vi "Client 1 JKI SM or SMO.vi"(4 "Enum 2":enum16{"SMO", "Stand Alone"}(ring)=enum."Stand Alone", 6 "Enum":enum16{"RemoteControl", "RemoteControl.STM"}(ring)=enum."RemoteControl.STM", 8 "error in (no error)":errorcluster, 10 "Message to Send":T1) -> (0 "error out":errorcluster, 1 "execution time (ms)":u32, 2 "Message Received":T1)   [LabVIEW 2016, in "RemoteControl.lvclass"]
uses:
  RemoteControl.lvclass
  <vilib>/JKI/JKI SMO/SMO/Typedefs/SMOState --Enum.ctl
  Typedefs/Message--Cluster.ctl
  RemoteControl.STM/RemoteControl.STM.lvclass
  C:/user/patrick/hg/levylab_util_remote/src/SMOs/RemoteControl/RemoteControl.lvclass
  <vilib>/JKI/JKI SMO/SMO/SMO.lvclass
  Typedefs/PrivateEvents--RemoteControl.SendMessageToProcess.ctl
  C:/Program Files (x86)/National Instruments/LabVIEW 2016/vi.lib/JKI/JKI SMO/SMO/SMO.lvclass
panel:
  out "# reads":i32
  out "send time":u32
  in  "timeout in ms (100)":i32=10
  in  "Send Message":bool
  in  "Stop":bool
  out "message backlog":i32
  out "messages received":i32
  out "messages sent":i32
  in  "Port":u32=6341
  in  "Address":string
  out "SMO State":T2
  # "Client 1"
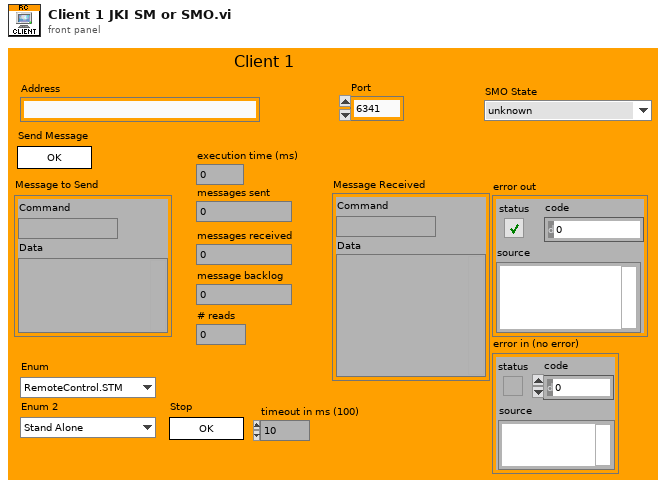
[diagram p1: front panel]
types:
  T1 = typedef "RemoteControl.lvclass/Message--Cluster.ctl" = cluster{"Command":string, "Data":variant}
  T2 = typedef "SMO.lvclass/SMOState --Enum.ctl" = enum16{"unknown", "Created", "Started", "Stopped"}
  T3 = enum32{"Invalid", "Standard", "Closed", "Hidden", "Minimized", "Maximized"}
  T4 = enum32{"invalid app kind", "Development System", "Run Time System", "Student Edition", "Embedded LabVIEW", "Evaluation", "Custom"}
  T5 = typedef "RemoteControl.lvclass/PrivateEvents--RemoteControl.SendMessageToProcess.ctl" = cluster{"Message":T1, "Message ID":u32}
  T6 = cluster{"Core":cluster{"Current VI Reference":refnum<vi>, "Close Panel on Exit?":bool}, "RemoteControl out":refnum<class "RemoteControl.lvclass">}
  T7 = cluster{"Current VI Reference":refnum<vi>, "Close Panel on Exit?":bool}
  T8 = typedef "SMO.lvclass/Public Events.ctl" = cluster{"Error":refnum<user-event>, "State":refnum<user-event>, "Reserve State":refnum<user-event>}
  T9 = typedef "RemoteControl.lvclass/PublicEvents--Cluster.ctl" = cluster{"SendMessageFromProcess":refnum<user-event>}
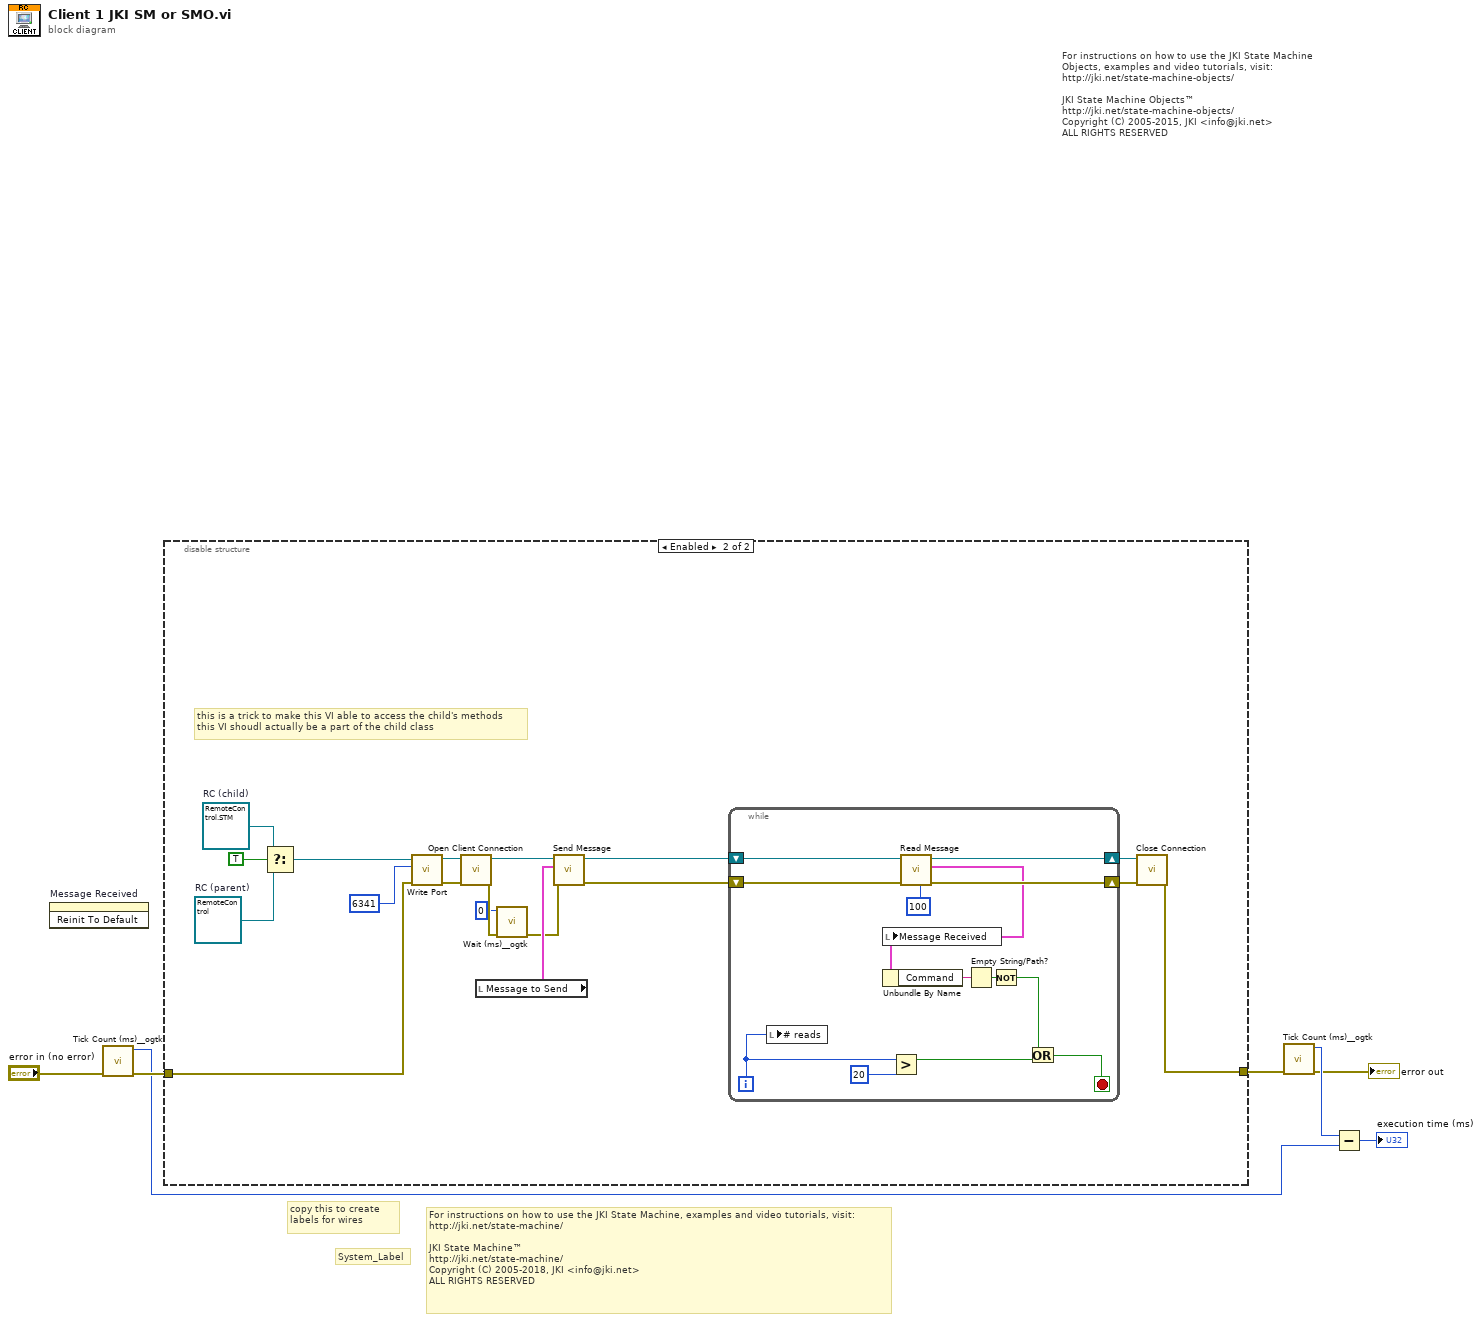
[diagram p0: block diagram]
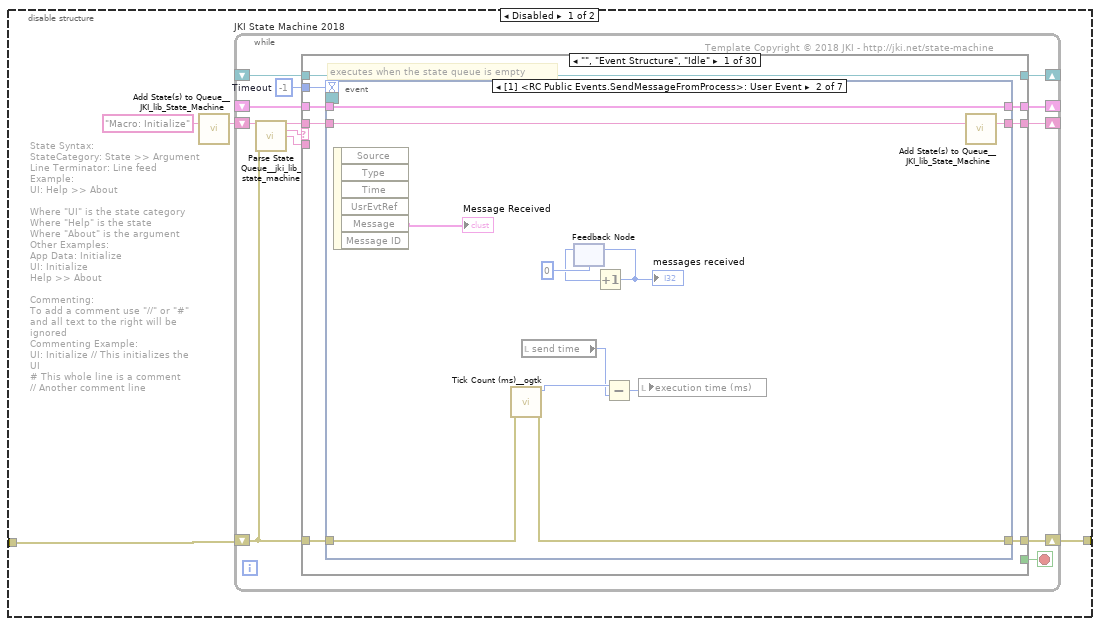
[diagram p2: hidden frame]
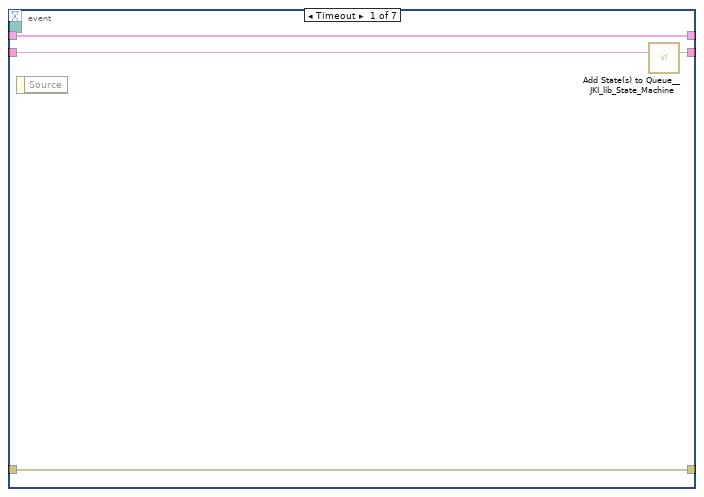
[diagram p3: hidden frame]
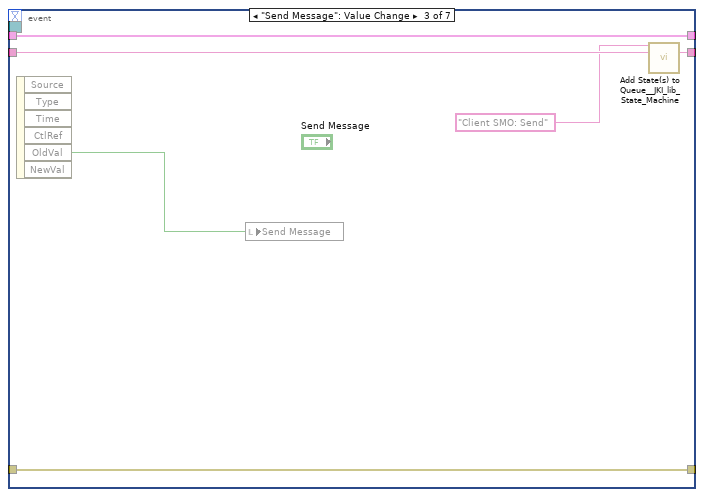
[diagram p4: hidden frame]
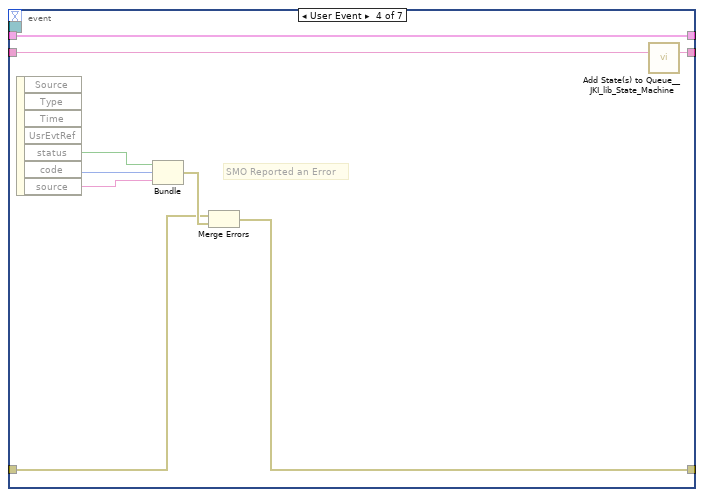
[diagram p5: hidden frame]
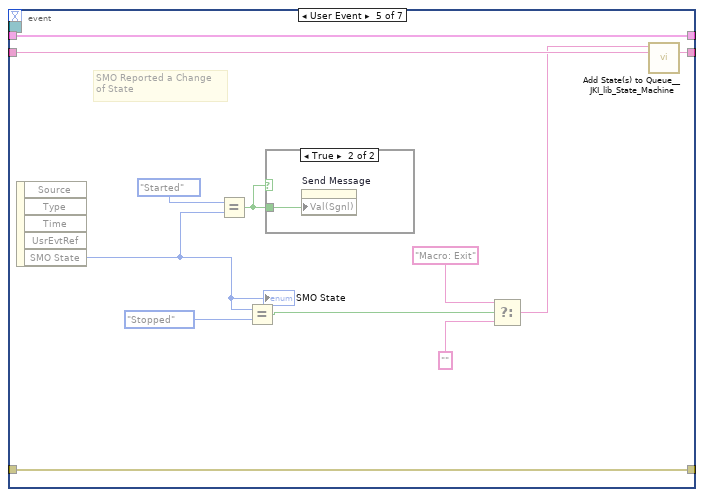
[diagram p6: hidden frame]
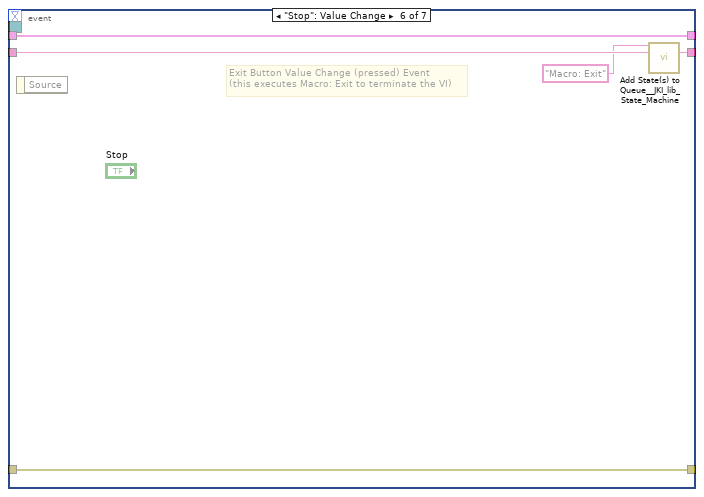
[diagram p8: hidden frame]
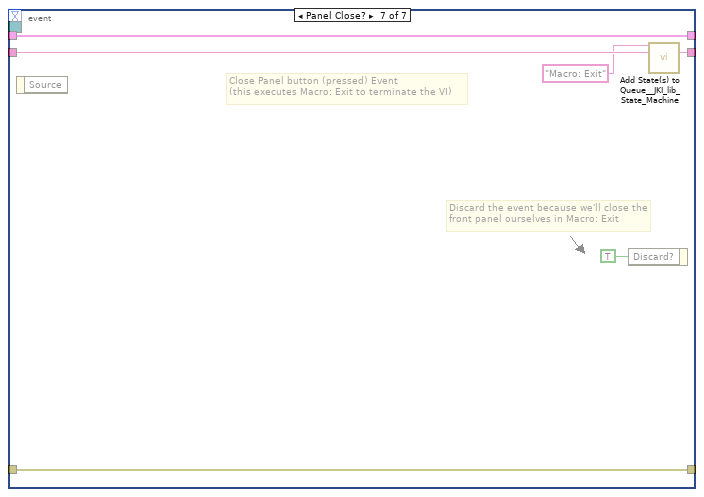
[diagram p9: hidden frame]
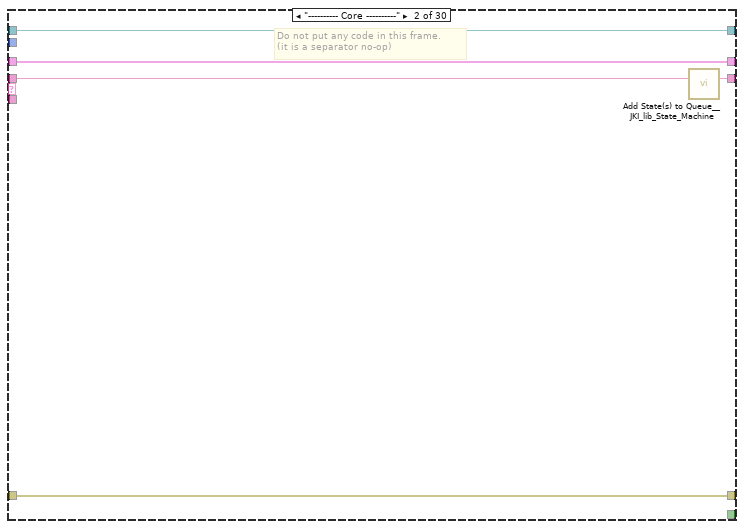
[diagram p10: hidden frame]
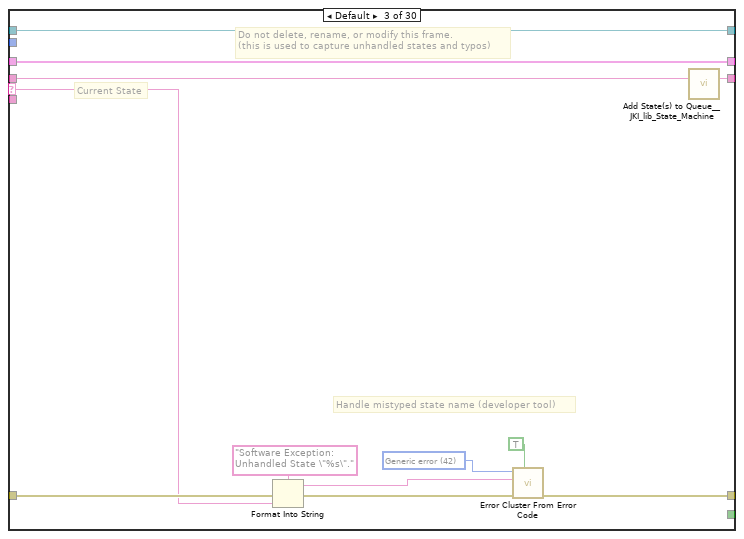
[diagram p11: hidden frame]
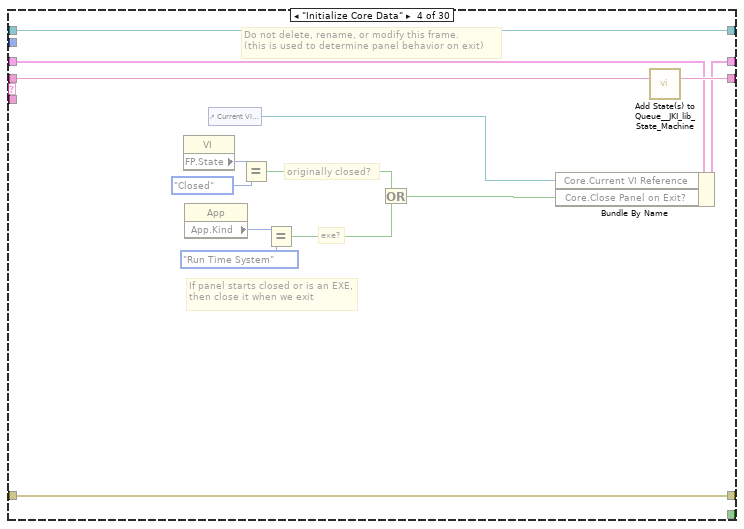
[diagram p12: hidden frame]
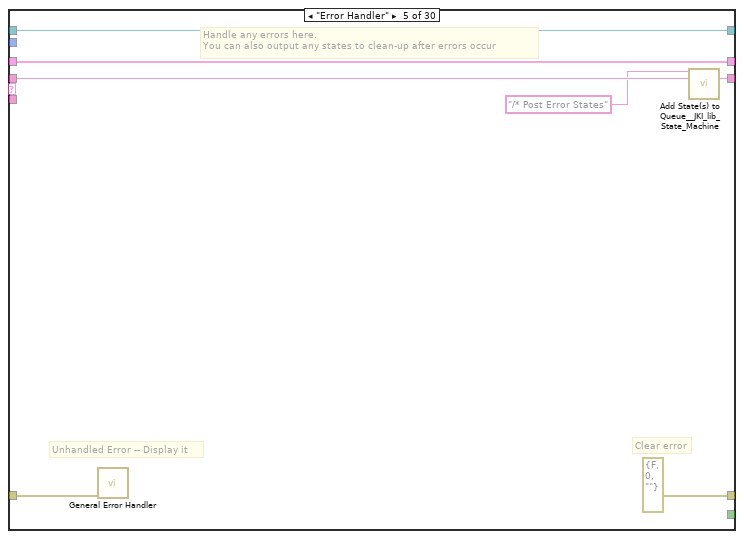
[diagram p13: hidden frame]
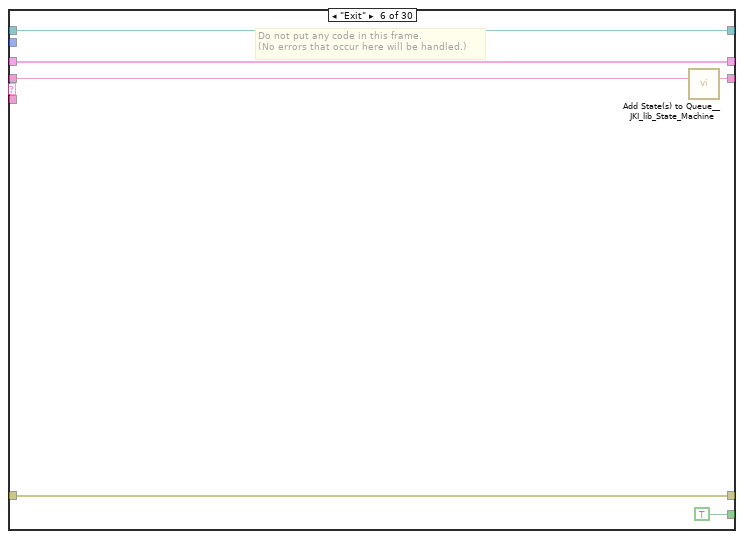
[diagram p14: hidden frame]
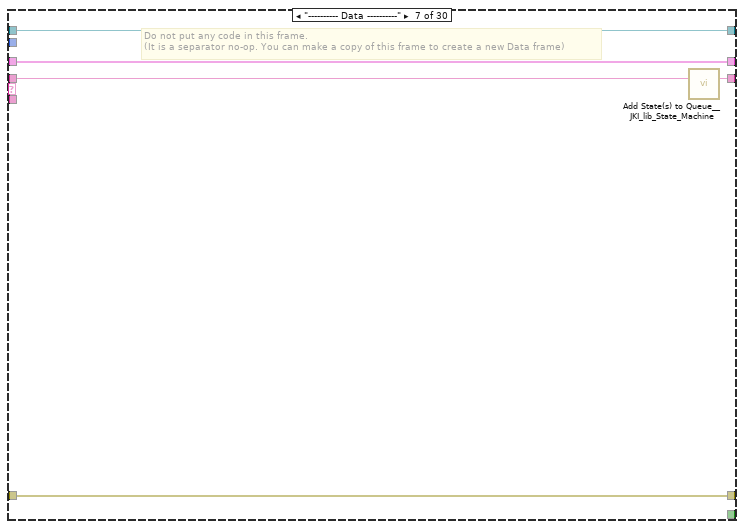
[diagram p15: hidden frame]
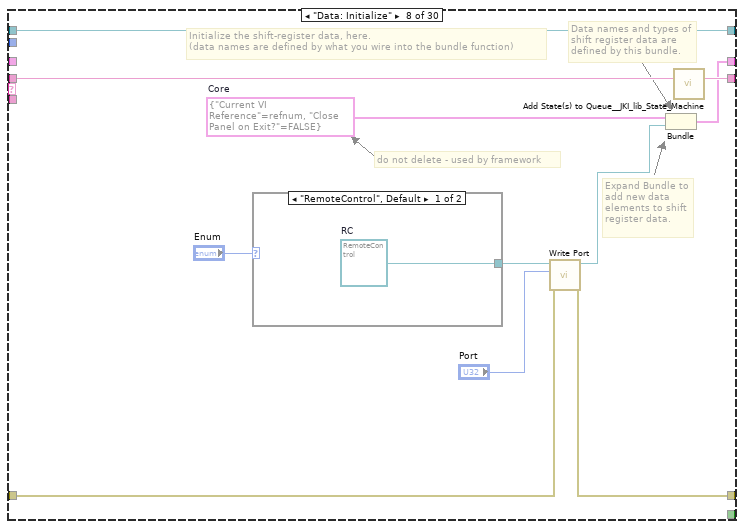
[diagram p16: hidden frame]
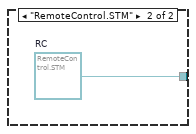
[diagram p17: hidden frame]
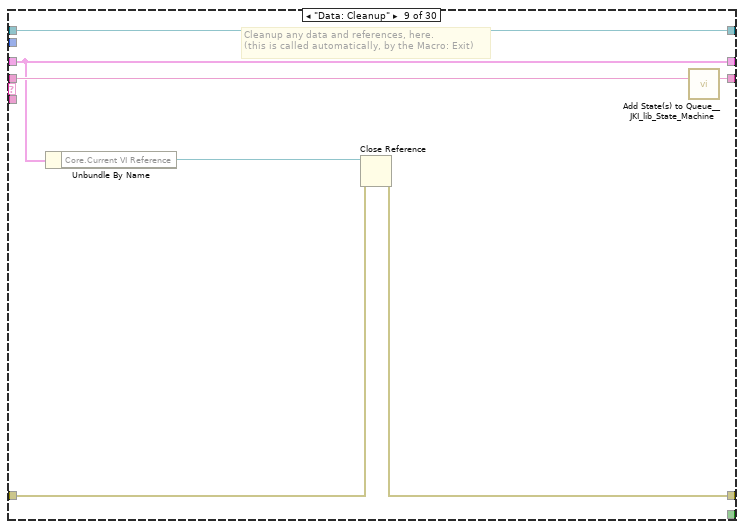
[diagram p18: hidden frame]
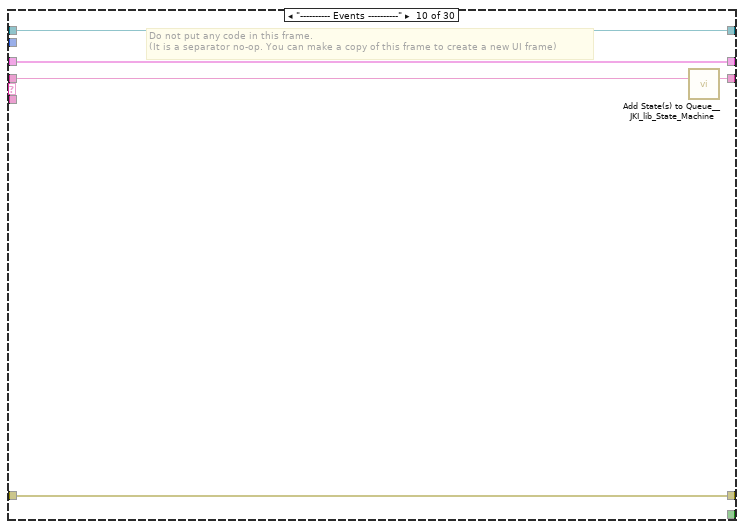
[diagram p19: hidden frame]
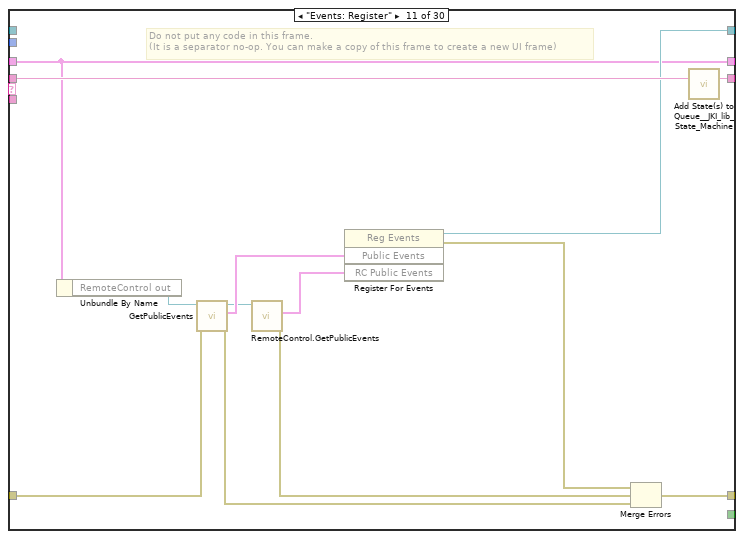
[diagram p20: hidden frame]
diagram:
  # "For instructions on how to use the JKI State Machine, examples and video tutorials, visit:\nhttp://jki.net/state-machine/\n\nJKI State Machine™\nhttp://jki.net/state-machine/\nCopyright (C) 2005-2018, JKI <info@jki.net>\nALL RIGHTS RESERVED"
  # "copy this to create labels for wires"
  # "System_Label"
  # "For instructions on how to use the JKI State Machine Objects, examples and video tutorials, visit:\nhttp://jki.net/state-machine-objects/\n\nJKI State Machine Objects™\nhttp://jki.net/state-machine-objects/\nCopyright (C) 2005-2015, JKI <info@jki.net>\nALL RIGHTS RESERVED"
  n1 = invoke on="Message Received" class="Clust (strict)" method="Reinit To Default"() -> ()  [unwired: 3 in, 3 out]
  n2 = call <userlib>:"Tick Count (ms)__ogtk.vi"("error in (no error)"="error in (no error)") -> ("error out"=w6:errorcluster, "millisecond timer value"=w1:u32)  [unwired: 9 in]
  n3 = disable-structure shown="Enabled" {
    disable-tunnel: w6 -> [w9 w425]
    disable-tunnel: [w8 w424] -> w2
    frame Disabled {
      # "State Syntax:\nStateCategory: State >> Argument\nLine Terminator: Line feed\nExample:\nUI: Help >> About\n\nWhere \"UI\" is the state category\nWhere \"Help\" is the state\nWhere \"About\" is the argument\nOther Examples:\nApp Data: Initialize\nUI: Initialize\nHelp >> About\n\nCommenting:\nTo add a comment use \"//\" or \"#\" and all text to the right will be ignored\nCommenting Example:\nUI: Initialize // This initializes the UI\n# This whole line is a comment\n// Another comment line"
      n4 = call <vilib>:"Add State(s) to Queue__JKI_lib_State_Machine.vi"("State(s) in (\"\")"="Macro: Initialize") -> ("States Out"=w11:string)  [unwired: 14 in]
      n5 = while "JKI State Machine 2018" {
        shift-right: [w17] -> _
        shift-left: _ -> [w16]
        shift-right: [w20] -> w8
        shift-left: w9 -> [w14]
        shift-right: [w19] -> _
        shift-left: w11 -> [w21]
        shift-right: [w13] -> _
        shift-left: _ -> [w12]
        stop <- w18 stop-if-true
        w15 = -1  # Timeout
        # "Template Copyright © 2018 JKI - http://jki.net/state-machine"
        n6 = call <vilib>:"Parse State Queue__jki_lib_state_machine.vi"("State Queue"=w21, "Error In (no error)"=w14) -> ("Remaining States"=w23:string, "Current State"=w24:string, "Arguments"=w22:string)  [unwired: 11 in]
        n7 = case shown="\"\", \"Event Structure\", \"Idle\"" w24 {
          selector: w24 -> [_ _ w94 _ _ _ _ _ _ _ _ _ _ _ _ _ _ _ _ _ _ _ _ _ _ _ _ _ _ _]
          tunnel: w23 -> [w32 w92 w98 w118 w125 w131 w136 w147 w156 w161 w174 w180 w185 w190 w197 w209 w279 w286 w299 w304 w317 w326 w343 w352 w359 w364 w373 w385 w396 w418]
          tunnel: w22 -> [_ _ _ _ _ _ _ _ _ _ _ _ _ _ w192 w203 _ _ _ _ _ _ _ _ _ _ _ _ _ _]
          tunnel: w16 -> [w30 w89 w96 w111 w122 w129 w133 _ w151 w158 w164 w178 w182 w188 w195 w205 w276 w283 w296 w301 w314 w323 w340 w349 w353 w361 w370 w382 w393 w415]
          tunnel: [w29 w90 w100 w115 errorcluster {"status"=FALSE, "code"=0, "source"=""} ("error out") w128 w134 w138 w152 w159 w170 w175 w183 w187 w193 w206 w277 w284 w297 w302 w305 w320 w338 w346 w355 w362 w365 w378 w387 w410] -> w20
          tunnel: w14 -> [w28 w90 w99 w115 w121 w128 w134 w139 w153 w159 w171 w176 w183 w187 w194 w207 w277 w284 w297 w302 w307 w321 w329 w347 w356 w362 w366 w376 w388 w412]
          tunnel: [w31 w91 w97 w117 w124 w130 w135 w146 w155 w160 w173 w179 w184 w189 w196 w208 w278 w285 w298 w303 w316 w325 w342 w351 w358 w363 w372 w384 w395 w417] -> w19
          tunnel: [_ _ _ _ _ TRUE _ _ _ _ _ _ _ _ _ _ _ _ _ _ _ _ _ _ _ _ _ _ _ _] -> w18
          tunnel: [w27 w89 w96 w116 w122 w129 w133 w145 w151 w158 w164 w178 w182 w188 w195 w205 w276 w283 w296 w301 w313 w322 w340 w348 w353 w361 w369 w381 w392 w414] -> w17
          tunnel: w15 -> [w26 _ _ _ _ _ _ _ _ _ _ _ _ _ _ _ _ _ _ _ _ _ _ _ _ _ _ _ _ _]
          tunnel: [w25 w88 w93 w105 w119 w126 w132 w143 w150 w157 w172 w177 w181 w186 w191 w202 w275 w282 w289 w300 w315 w324 w341 w350 w357 w360 w371 w383 w394 w416] -> w13
          tunnel: w12 -> [w25 w88 w93 w105 w119 w126 w132 w143 w150 w157 _ w177 w181 w186 w191 w202 w275 w282 w289 w300 w315 w324 w341 w350 w357 w360 w371 w383 w394 w416]
          frame "", "Event Structure", "Idle" {
            # "executes when the state queue is empty"
            n8 = event shown="[1] <RC Public Events.SendMessageFromProcess>: User Event" {
              selector: w25 -> [_ _ _ _ _ _ _]
              dyn-events: _ -> [_ _ _ _ _ _ _]
              timeout: w26 -> [_ _ _ _ _ _ _]
              tunnel: w32 -> [w36 w48 w54 w63 w75 w81 w87]
              tunnel: [w35 w47 w53 w62 w74 w80 w86] -> w31
              tunnel: w30 -> [w33 w46 w51 w61 w72 w78 w84]
              tunnel: [w34 w40 w52 w55 w73 w79 w85] -> w29
              tunnel: w28 -> [w34 w41 w52 w56 w73 w79 w85]
              tunnel: [w33 w46 w51 w61 w72 w78 w84] -> w27
              event Timeout {
                n9 = event-data() -> ()  [unwired: 1 in, 1 out]
                n10 = call <vilib>:"Add State(s) to Queue__JKI_lib_State_Machine.vi"("State(s) in (\"\")"=w36) -> ("States Out"=w35:string)  [unwired: 14 in]
              }
              event User Event {
                n11 = event-data() -> ("Message"=→"Message Received":T1)  [unwired: 1 in, 5 out]
                n12 = call <userlib>:"Tick Count (ms)__ogtk.vi"("error in (no error)"=w41) -> ("error out"=w40:errorcluster, "millisecond timer value"=w39:u32)  [unwired: 9 in]
                n13 = local read "send time"() -> (w38:u32)
                n14 = feedback #1(0) -> (w43:i32)
                n15 = Increment(x=w43) -> (x+1=w42:i32)
                "messages received" <- w42
                n16 = feedback-in #1(w42) -> ()
                n17 = Subtract(x=w39, y=w38) -> (x-y=w37:u32)
                n18 = local write "execution time (ms)"(w37) -> ()
                n19 = call <vilib>:"Add State(s) to Queue__JKI_lib_State_Machine.vi"("State(s) in (\"\")"=w48) -> ("States Out"=w47:string)  [unwired: 14 in]
              }
              event "Send Message": Value Change {
                n20 = event-data() -> ("OldVal"=w49:bool)  [unwired: 1 in, 5 out]
                n21 = local write "Send Message"(w49) -> ()
                n22 = call <vilib>:"Add State(s) to Queue__JKI_lib_State_Machine.vi"("State(s) in Front (\"\")"="Client SMO: Send" ("State(s) in Front (\"\")"), "State(s) in (\"\")"=w54) -> ("States Out"=w53:string)  [unwired: 13 in]
              }
              event User Event {
                # "SMO Reported an Error"
                n23 = event-data() -> ("status"=w60:bool, "code"=w59:i32, "source"=w58:string)  [unwired: 1 in, 4 out]
                n24 = Bundle("status"=w60, "code"=w59, "source"=w58) -> (w57:errorcluster)  [unwired: 1 in]
                n25 = Merge Errors(w56, w57) -> (w55:errorcluster)
                n26 = call <vilib>:"Add State(s) to Queue__JKI_lib_State_Machine.vi"("State(s) in (\"\")"=w63) -> ("States Out"=w62:string)  [unwired: 14 in]
              }
              event User Event {
                # "SMO Reported a Change\nof State"
                n27 = event-data() -> ("SMO State"=w66:T2)  [unwired: 1 in, 4 out]
                "SMO State" <- w66
                n28 = Equal?(x=SMOState_--Enum."Started" ("y"), y=w66) -> (x = y?=w64:bool)
                n29 = Equal?(x=w66, y=SMOState_--Enum."Stopped") -> (x = y?=w70:bool)
                n30 = case shown="True" w64 {
                  tunnel: w64 -> [_ w76]
                  frame False {
                  }
                  frame True {
                    n31 = property on="Send Message" class="Bool (strict)"("Val(Sgnl)"=w76) -> ()  [unwired: 2 in, 2 out]
                  }
                }
                n32 = Select(t="Macro: Exit" ("State(s) in Front (\"\")"), s=w70, f="" ("State(s) in Front (\"\")")) -> (s? t:f=w69:string)
                n33 = call <vilib>:"Add State(s) to Queue__JKI_lib_State_Machine.vi"("State(s) in Front (\"\")"=w69, "State(s) in (\"\")"=w75) -> ("States Out"=w74:string)  [unwired: 13 in]
              }
              event "Stop": Value Change {
                # "Exit Button Value Change (pressed) Event\n(this executes Macro: Exit to terminate the VI)"
                n34 = event-data() -> ()  [unwired: 1 in, 1 out]
                n35 = call <vilib>:"Add State(s) to Queue__JKI_lib_State_Machine.vi"("State(s) in Front (\"\")"="Macro: Exit", "State(s) in (\"\")"=w81) -> ("States Out"=w80:string)  [unwired: 13 in]
              }
              event Panel Close? {
                # "Discard the event because we'll close the front panel ourselves in Macro: Exit"
                # "Close Panel button (pressed) Event\n(this executes Macro: Exit to terminate the VI)"
                n36 = event-data() -> ()  [unwired: 1 in, 1 out]
                n37 = event-data("Discard?"=TRUE) -> ()  [unwired: 1 in, 1 out]
                n38 = call <vilib>:"Add State(s) to Queue__JKI_lib_State_Machine.vi"("State(s) in Front (\"\")"="Macro: Exit", "State(s) in (\"\")"=w87) -> ("States Out"=w86:string)  [unwired: 13 in]
              }
            }
          }
          frame "---------- Core ----------" {
            # "Do not put any code in this frame.\n(it is a separator no-op)"
            n39 = call <vilib>:"Add State(s) to Queue__JKI_lib_State_Machine.vi"("State(s) in (\"\")"=w92) -> ("States Out"=w91:string)  [unwired: 14 in]
          }
          frame Default {
            w103 = 42 items=["No error", "Argument error", "Memory is full", "Out of zone", "End of file", "File already open", "Generic file I/O error", "File not found", "File permission error", "Disk is full", "Duplicate path", "Too many files open", "System feature not enabled", "Resource file not found", "Cannot add resource", "Resource not found", "Image not found", "Image memory error", "Pen does not exist", "Config type invalid", "Config token not found", "Config parse error", "Config memory error", "Bad external code format", "Bad external code offset", "External code not present", "Null window", "Destroy window error", "Null menu", "Print aborted", "Bad print record", "Print driver error", "Windows error during printing", "Memory error during printing", "Print dialog error", "Generic print error", "Invalid device refnum", "Device not found", "Device parameter error", "Device unit error", "Cannot open device", "Device call aborted", "Generic error", "Cancelled by user", "Object ID too low", "Object ID too high", "Object not in heap", "Unknown heap", "Unknown object (invalid DefProc)", "Unknown object (DefProc not in table)", "Message out of range", "Invalid (null) method", "Unknown message", "Manager call not supported", "Bad address", "Network operation in progress", "Network operation timed out", "Connection is busy", "Network attribute not supported", "Network error", "Address in use", "System out of memory", "Connection aborted", "Connection refused", "Not connected", "Already connected", "Connection closed", "Initialization error (interapplication manager)", "Bad occurrence", "Wait on unbound occurrence handler", "Occurrence queue overflow", "Datalog type conflict", "Unused", "Unrecognized type (interapplication manager)", "Memory corrupt", "Failed to make temporary DLL", "Old CIN version", "Drag socket not found", "Failed to load drop-object", "Failed to register OLE object", "Failed to release OLE object", "Format specifier type mismatch", "Unknown format specifier", "Too few format specifiers", "Too many format specifiers", "Scan failed", "Newer CIN version", "Error converting to variant", "Runtime menu error", "Password tampered", "Variant attribute not found", "Incompatible variant data type", "Event data is not available", "Event Store is not present", "Occurrence is not found", "Event Queue is not created", "Event info is not available", "Refnum passed is NULL", "Error retrieving Class GUID", "Error retrieving CoClass GUID", "Error retrieving TypeLib GUID.", "Bad built application magic bytes.", "Specific driver is different from the specific driver associated with the Logical Name.", "There is no session opened to the class driver.", "Max Error", "MAX - Error with config objects", "MAX - Error loading configuration", "MAX - Group not supported"]
            # "Current State"
            # "Do not delete, rename, or modify this frame.\n(this is used to capture unhandled states and typos)"
            # "Handle mistyped state name (developer tool)"
            n40 = Format Into String(format string="Software Exception: Unhandled State \"%s\"." ("message"), error in=w99, w94) -> (resulting string=w102:string, error out=w101:errorcluster)  [unwired: 1 in]
            n41 = call <vilib>:"Error Cluster From Error Code.vi"("show call chain? (False)"=TRUE, "error in (no error)"=w101, "error message (\"\")"=w102, "error code (0)"=w103) -> ("error out"=w100:errorcluster)  [unwired: 5 in]
            n42 = call <vilib>:"Add State(s) to Queue__JKI_lib_State_Machine.vi"("State(s) in (\"\")"=w98) -> ("States Out"=w97:string)  [unwired: 14 in]
          }
          frame "Initialize Core Data" {
            # "Do not delete, rename, or modify this frame.\n(this is used to determine panel behavior on exit)"
            # "originally closed?"
            # "exe?"
            # "If panel starts closed or is an EXE, then close it when we exit"
            n43 = property class="VI"() -> ("FP.State"=w108:T3)  [unwired: 2 in, 2 out]
            n44 = property class="App"() -> ("App.Kind"=w114:T4)  [unwired: 2 in, 2 out]
            n45 = control-ref of="Current VI Reference"() -> (w109:refnum<vi>)
            n46 = Equal?(x=w108, y=T3."Closed" ("Front Panel Window:State")) -> (x = y?=w106:bool)
            n47 = Equal?(x=w114, y=T4."Run Time System" ("Application:Kind")) -> (x = y?=w112:bool)
            n48 = Or(x=w106, y=w112) -> (x .or. y?=w110:bool)
            n49 = Bundle By Name(cluster=w111, "Core.Current VI Reference"=w109, "Core.Close Panel on Exit?"=w110) -> (w116:T6)
            n50 = call <vilib>:"Add State(s) to Queue__JKI_lib_State_Machine.vi"("State(s) in (\"\")"=w118) -> ("States Out"=w117:string)  [unwired: 14 in]
          }
          frame "Error Handler" {
            # "Unhandled Error -- Display it"
            # "Handle any errors here.\nYou can also output any states to clean-up after errors occur"
            # "Clear error"
            n51 = call <vilib>:"General Error Handler.vi"("error in (no error)"=w121) -> ()  [unwired: 10 in, 5 out]
            n52 = call <vilib>:"Add State(s) to Queue__JKI_lib_State_Machine.vi"("State(s) in Front (\"\")"="/* Post Error States", "State(s) in (\"\")"=w125) -> ("States Out"=w124:string)  [unwired: 13 in]
          }
          frame "Exit" {
            # "Do not put any code in this frame.\n(No errors that occur here will be handled.)"
            n53 = call <vilib>:"Add State(s) to Queue__JKI_lib_State_Machine.vi"("State(s) in (\"\")"=w131) -> ("States Out"=w130:string)  [unwired: 14 in]
          }
          frame "---------- Data ----------" {
            # "Do not put any code in this frame.\n(It is a separator no-op. You can make a copy of this frame to create a new Data frame)"
            n54 = call <vilib>:"Add State(s) to Queue__JKI_lib_State_Machine.vi"("State(s) in (\"\")"=w136) -> ("States Out"=w135:string)  [unwired: 14 in]
          }
          frame "Data: Initialize" {
            w144 = T7 {"Current VI Reference"=refnum, "Close Panel on Exit?"=FALSE}  # Core
            # "do not delete - used by framework"
            # "Expand Bundle to add new data elements to shift register data."
            # "Data names and types of shift register data are defined by this bundle."
            # "Initialize the shift-register data, here.\n(data names are defined by what you wire into the bundle function)"
            n55 = case shown="\"RemoteControl\", Default" "Enum" {
              tunnel: [w148 w149] -> w141
              frame "RemoteControl", Default {
                w148 = refnum<class "RemoteControl.lvclass"> refnum  # RC
              }
              frame "RemoteControl.STM" {
                w149 = refnum<class "RemoteControl.STM.lvclass"> refnum  # RC
              }
            }
            n56 = call-dynamic "Write Port.vi"("error in (no error)"=w139, "Port"="Port", "RemoteControl in"=w141) -> ("error out"=w138:errorcluster, "RemoteControl out"=w140:refnum<class "RemoteControl.lvclass">)  [unwired: 7 in]
            n57 = Bundle("Core"=w144, "RemoteControl out"=w140) -> (w145:T6)  [unwired: 1 in]
            n58 = call <vilib>:"Add State(s) to Queue__JKI_lib_State_Machine.vi"("State(s) in (\"\")"=w147) -> ("States Out"=w146:string)  [unwired: 14 in]
          }
          frame "Data: Cleanup" {
            # "Cleanup any data and references, here.\n(this is called automatically, by the Macro: Exit)"
            n59 = Unbundle By Name(w151) -> ("Core.Current VI Reference"=w154:refnum<vi>)
            n60 = Close Reference(reference=w154, error in (no error)=w153) -> (error out=w152:errorcluster)
            n61 = call <vilib>:"Add State(s) to Queue__JKI_lib_State_Machine.vi"("State(s) in (\"\")"=w156) -> ("States Out"=w155:string)  [unwired: 14 in]
          }
          frame "---------- Events ----------" {
            # "Do not put any code in this frame.\n(It is a separator no-op. You can make a copy of this frame to create a new UI frame)"
            n62 = call <vilib>:"Add State(s) to Queue__JKI_lib_State_Machine.vi"("State(s) in (\"\")"=w161) -> ("States Out"=w160:string)  [unwired: 14 in]
          }
          frame "Events: Register" {
            # "Do not put any code in this frame.\n(It is a separator no-op. You can make a copy of this frame to create a new UI frame)"
            n63 = Unbundle By Name(w164) -> ("RemoteControl out"=w163:refnum<class "RemoteControl.lvclass">)
            n64 = call <vilib>:"GetPublicEvents.vi"("error in (no error)"=w171, "SMO"=w163) -> ("error out"=w167:errorcluster, "Public Events"=w169:T8, "SMO out"=w162:refnum<class "RemoteControl.lvclass">)  [unwired: 7 in]
            n65 = call "RemoteControl.GetPublicEvents.vi"("RemoteControl"=w162) -> ("error out"=w166:errorcluster, "RC Public Events"=w168:T9)  [unwired: 8 in, 1 out]
            n66 = register-events(w169, w168) -> (reference out=w172:refnum<event-registration>, error out=w165:errorcluster)  [unwired: 2 in]
            n67 = Merge Errors(w165, w166, w167) -> (w170:errorcluster)
            n68 = call <vilib>:"Add State(s) to Queue__JKI_lib_State_Machine.vi"("State(s) in (\"\")"=w174) -> ("States Out"=w173:string)  [unwired: 14 in]
          }
          frame "Events: Unregister" {
            # "Do not put any code in this frame.\n(It is a separator no-op. You can make a copy of this frame to create a new UI frame)"
            n69 = Unregister For Events(event registration refnum=w177, error in=w176) -> (error out=w175:errorcluster)
            n70 = call <vilib>:"Add State(s) to Queue__JKI_lib_State_Machine.vi"("State(s) in (\"\")"=w180) -> ("States Out"=w179:string)  [unwired: 14 in]
          }
          frame "---------- UI ----------" {
            # "Do not put any code in this frame.\n(It is a separator no-op. You can make a copy of this frame to create a new UI frame)"
            n71 = call <vilib>:"Add State(s) to Queue__JKI_lib_State_Machine.vi"("State(s) in (\"\")"=w185) -> ("States Out"=w184:string)  [unwired: 14 in]
          }
          frame "UI: Initialize" {
            # "Initialize the User Interface, here.\n(this is called automatically, by the Macro: Init)"
            n72 = invoke on="error out" class="Clust (strict)" method="Reinit To Default"() -> ()  [unwired: 3 in, 3 out]
            n73 = invoke on="SMO State" class="Enum (strict)" method="Reinit To Default"() -> ()  [unwired: 3 in, 3 out]
            n74 = call <vilib>:"Add State(s) to Queue__JKI_lib_State_Machine.vi"("State(s) in (\"\")"=w190) -> ("States Out"=w189:string)  [unwired: 14 in]
          }
          frame "UI: Cursor Set" {
            # "Argument"
            # "Set and Unset Cursor Busy.\n(Usage: \"UI: Cursor Set >> Busy|Idle\")"
            n75 = case shown="\"Idle\", Default" w192 {
              tunnel: w194 -> [w199 w201]
              tunnel: [w198 w200] -> w193
              frame "Idle", Default {
                n76 = call <vilib>:"Unset Busy.vi"("error in (no error)"=w199) -> ("error out"=w198:errorcluster)  [unwired: 10 in]
              }
              frame "Busy" {
                n77 = call <vilib>:"Set Busy.vi"("error in (no error)"=w201) -> ("error out"=w200:errorcluster)  [unwired: 9 in, 1 out]
              }
            }
            n78 = call <vilib>:"Add State(s) to Queue__JKI_lib_State_Machine.vi"("State(s) in (\"\")"=w197) -> ("States Out"=w196:string)  [unwired: 14 in]
          }
          frame "UI: Front Panel State" {
            # "Argument"
            # "Set Front Panel Open or Closed\n(Usage: \"UI: Front Panel State >> Open|Close\")"
            n79 = Unbundle By Name(w205) -> ("Core.Current VI Reference"=w204:refnum<vi>)
            n80 = case shown="\"Minimize\", \"Minimized\"" w203 {
              tunnel: w207 -> [w215 w230 w241 w254 w267]
              tunnel: [w217 w231 w243 w256 w269] -> w206
              tunnel: w204 -> [w216 w228 w242 w255 w268]
              frame "Open", "Standard", Default {
                w210 = T3."Standard" ("State")
                n81 = property class="VI"(reference=w216, error in=w215) -> (reference out=w213:refnum<vi>, error out=w214:errorcluster, "FP.State"=w212:T3)
                n82 = Not Equal?(x=w212, y=w210) -> (x != y?=w211:bool)
                n83 = case shown="True" w211 {
                  tunnel: [w221 w223] -> w217
                  tunnel: w214 -> [w220 w223]
                  tunnel: w213 -> [w219 _]
                  tunnel: w210 -> [w218 _]
                  frame True {
                    n84 = invoke class="VI" method="FP.Open"(reference=w219, error in=w220, "Activate"=TRUE, "State"=w218) -> (error out=w221:errorcluster)  [unwired: 1 in, 4 out]
                  }
                  frame False {
                  }
                }
              }
              frame "Close", "Closed" {
                n85 = property class="VI"(reference=w228, error in=w230) -> (reference out=w227:refnum<vi>, error out=w229:errorcluster, "FP.State"=w225:T3)
                n86 = Not Equal?(x=w225, y=T3."Closed" ("Front Panel Window:State")) -> (x != y?=w224:bool)
                n87 = case shown="True" w224 {
                  tunnel: [w232 w235] -> w231
                  tunnel: w229 -> [w232 w234]
                  tunnel: w227 -> [_ w233]
                  frame False {
                  }
                  frame True {
                    n88 = invoke class="VI" method="FP.Close"(reference=w233, error in=w234) -> (error out=w235:errorcluster)  [unwired: 1 in, 2 out]
                  }
                }
              }
              frame "Hidden", "Hide" {
                w236 = T3."Hidden" ("State")
                n89 = property class="VI"(reference=w242, error in=w241) -> (reference out=w239:refnum<vi>, error out=w240:errorcluster, "FP.State"=w238:T3)
                n90 = Not Equal?(x=w238, y=w236) -> (x != y?=w237:bool)
                n91 = case shown="True" w237 {
                  tunnel: [w247 w248] -> w243
                  tunnel: w240 -> [w246 w248]
                  tunnel: w239 -> [w245 _]
                  tunnel: w236 -> [w244 _]
                  frame True {
                    n92 = invoke class="VI" method="FP.Open"(reference=w245, error in=w246, "State"=w244) -> (error out=w247:errorcluster)  [unwired: 2 in, 4 out]
                  }
                  frame False {
                  }
                }
              }
              frame "Minimize", "Minimized" {
                w249 = T3."Minimized" ("State")
                n93 = property class="VI"(reference=w255, error in=w254) -> (reference out=w252:refnum<vi>, error out=w253:errorcluster, "FP.State"=w251:T3)
                n94 = Not Equal?(x=w251, y=w249) -> (x != y?=w250:bool)
                n95 = case shown="True" w250 {
                  tunnel: [w260 w261] -> w256
                  tunnel: w253 -> [w259 w261]
                  tunnel: w252 -> [w258 _]
                  tunnel: w249 -> [w257 _]
                  frame True {
                    n96 = invoke class="VI" method="FP.Open"(reference=w258, error in=w259, "State"=w257) -> (error out=w260:errorcluster)  [unwired: 2 in, 4 out]
                  }
                  frame False {
                  }
                }
              }
              frame "Maximize", "Maximized" {
                w262 = T3."Maximized" ("State")
                n97 = property class="VI"(reference=w268, error in=w267) -> (reference out=w265:refnum<vi>, error out=w266:errorcluster, "FP.State"=w264:T3)
                n98 = Not Equal?(x=w264, y=w262) -> (x != y?=w263:bool)
                n99 = case shown="True" w263 {
                  tunnel: [w273 w274] -> w269
                  tunnel: w266 -> [w272 w274]
                  tunnel: w265 -> [w271 _]
                  tunnel: w262 -> [w270 _]
                  frame True {
                    n100 = invoke class="VI" method="FP.Open"(reference=w271, error in=w272, "State"=w270) -> (error out=w273:errorcluster)  [unwired: 2 in, 4 out]
                  }
                  frame False {
                  }
                }
              }
            }
            n101 = call <vilib>:"Add State(s) to Queue__JKI_lib_State_Machine.vi"("State(s) in (\"\")"=w209) -> ("States Out"=w208:string)  [unwired: 14 in]
          }
          frame "---------- Macro ----------" {
            # "Do not put any code in this frame.\n(It is a separator no-op. You can make a copy of this frame to create a new Macro frame)"
            n102 = call <vilib>:"Add State(s) to Queue__JKI_lib_State_Machine.vi"("State(s) in (\"\")"=w279) -> ("States Out"=w278:string)  [unwired: 14 in]
          }
          frame "Macro: Initialize" {
            # "Initialization Macro\n(This is called once, when the VI starts)"
            n103 = case shown="\"Stand Alone\"" "Enum 2" {
              tunnel: ["Data: Initialize\nInitialize Core Data\nClient SMO: Create\nEvents: Register\nClient SMO: Start\nUI: Initialize\nUI: Front Panel State >> Open" "Data: Initialize\nInitialize Core Data\nClient: Open\nClient: Write\nClient: Read\nClient: Close\nData: Cleanup\nExit"] -> w280
              frame "SMO", Default {
              }
              frame "Stand Alone" {
              }
            }
            n104 = call <vilib>:"Add State(s) to Queue__JKI_lib_State_Machine.vi"("State(s) in Front (\"\")"=w280, "State(s) in (\"\")"=w286) -> ("States Out"=w285:string)  [unwired: 13 in]
          }
          frame "Macro: Exit" {
            # "Exit Macro\n(This is called once, when the VI exits)"
            n105 = Unbundle By Name(w296) -> ("Core.Close Panel on Exit?"=w295:bool)
            n106 = Select(t="UI: Front Panel State >> Close", s=w295, f="") -> (s? t:f=w292:string)
            n107 = call <vilib>:"Add State(s) to Queue__JKI_lib_State_Machine.vi"("State(s) in (\"\")"=w292, "State(s) at Back (\"\")"="Client SMO: Stop\nClient SMO: Destroy\nData: Cleanup\nEvents: Unregister\nExit") -> ("States Out"=w290:string)  [unwired: 13 in]
            n108 = call <vilib>:"Add State(s) to Queue__JKI_lib_State_Machine.vi"("State(s) in Front (\"\")"=w290, "State(s) in (\"\")"=w299) -> ("States Out"=w298:string)  [unwired: 13 in]
          }
          frame "---------- Client SMO ----------" {
            # "Template Separator\n(You can make a copy of, or modify, this frame)"
            n109 = call <vilib>:"Add State(s) to Queue__JKI_lib_State_Machine.vi"("State(s) in (\"\")"=w304) -> ("States Out"=w303:string)  [unwired: 14 in]
          }
          frame "Client SMO: Create" {
            # "Your code here.\n(You can make a copy of, or modify, this frame)"
            n110 = Unbundle By Name(w314) -> ("RemoteControl out"=w311:refnum<class "RemoteControl.lvclass">)
            n111 = call-dynamic "Read Port.vi"("error in (no error)"=w307, "RemoteControl in"=w311) -> ("error out"=w308:errorcluster, "Port"=w309:u16, "RemoteControl out"=w310:refnum<class "RemoteControl.lvclass">)  [unwired: 7 in]
            n112 = call-dynamic "Create RC Client.vi"("error in (no error)"=w308, "Port"=w309, "Address"="Address", "RemoteControl in"=w310) -> ("error out"=w305:errorcluster, "RemoteControl out"=w312:refnum<class "RemoteControl.lvclass">)  [unwired: 6 in]
            n113 = Bundle By Name(cluster=w314, "RemoteControl out"=w312) -> (w313:T6)
            n114 = call <vilib>:"Add State(s) to Queue__JKI_lib_State_Machine.vi"("State(s) in (\"\")"=w317) -> ("States Out"=w316:string)  [unwired: 14 in]
          }
          frame "Client SMO: Start" {
            # "Your code here.\n(You can make a copy of, or modify, this frame)"
            n115 = Unbundle By Name(w323) -> ("RemoteControl out"=w319:refnum<class "RemoteControl.lvclass">)
            n116 = call <vilib>:"Start.vi"("error in (no error)"=w321, "SMO"=w319) -> ("error out"=w320:errorcluster, "SMO out"=w318:refnum<class "RemoteControl.lvclass">)  [unwired: 8 in]
            n117 = Bundle By Name(cluster=w323, "RemoteControl out"=w318) -> (w322:T6)
            n118 = call <vilib>:"Add State(s) to Queue__JKI_lib_State_Machine.vi"("State(s) in (\"\")"=w326) -> ("States Out"=w325:string)  [unwired: 14 in]
          }
          frame "Client SMO: Send" {
            n119 = Unbundle By Name(w340) -> ("RemoteControl out"=w339:refnum<class "RemoteControl.lvclass">)
            n120 = Bundle By Name(cluster=T5 {"Message"={"Command"="", "Data"=variant(bool FALSE)}, "Message ID"=0} ("SendMessgaeToProcess"), "Message"="Message to Send") -> (w336:T5)
            n121 = call <userlib>:"Tick Count (ms)__ogtk.vi"("error in (no error)"=w329) -> ("error out"=w328:errorcluster, "millisecond timer value"=→"send time":u32)  [unwired: 9 in]
            n122 = call "RemoteControl.SendMessageToProcess.vi"("error in (no error)"=w328, "SendMessgaeToProcess"=w336, "RemoteControl"=w339) -> ("error out"=w338:errorcluster)  [unwired: 7 in, 1 out]
            n123 = feedback #2(0) -> (w331:i32)
            n124 = local read "messages received"() -> (w334:i32)
            n125 = Increment(x=w331) -> (x+1=w333:i32)
            "messages sent" <- w333
            n126 = feedback-in #2(w333) -> ()
            n127 = Subtract(x=w333, y=w334) -> (x-y=→"message backlog":i32)
            n128 = call <vilib>:"Add State(s) to Queue__JKI_lib_State_Machine.vi"("State(s) in (\"\")"=w343) -> ("States Out"=w342:string)  [unwired: 14 in]
          }
          frame "Client SMO: Stop" {
            # "Your code here.\n(You can make a copy of, or modify, this frame)"
            n129 = Unbundle By Name(w349) -> ("RemoteControl out"=w345:refnum<class "RemoteControl.lvclass">)
            n130 = call <vilib>:"Stop.vi"("error in (no error)"=w347, "SMO"=w345) -> ("error out"=w346:errorcluster, "SMO out"=w344:refnum<class "RemoteControl.lvclass">)  [unwired: 8 in]
            n131 = Bundle By Name(cluster=w349, "RemoteControl out"=w344) -> (w348:T6)
            n132 = call <vilib>:"Add State(s) to Queue__JKI_lib_State_Machine.vi"("State(s) in (\"\")"=w352) -> ("States Out"=w351:string)  [unwired: 14 in]
          }
          frame "Client SMO: Destroy" {
            # "Your code here.\n(You can make a copy of, or modify, this frame)"
            n133 = Unbundle By Name(w353) -> ("RemoteControl out"=w354:refnum<class "RemoteControl.lvclass">)
            n134 = call <vilib>:"Destroy.vi"("error in (no error)"=w356, "SMO"=w354) -> ("error out"=w355:errorcluster)  [unwired: 9 in]
            n135 = call <vilib>:"Add State(s) to Queue__JKI_lib_State_Machine.vi"("State(s) in (\"\")"=w359) -> ("States Out"=w358:string)  [unwired: 14 in]
          }
          frame "---------- Client ----------" {
            # "Template Separator\n(You can make a copy of, or modify, this frame)"
            n136 = call <vilib>:"Add State(s) to Queue__JKI_lib_State_Machine.vi"("State(s) in (\"\")"=w364) -> ("States Out"=w363:string)  [unwired: 14 in]
          }
          frame "Client: Open" {
            # "Your code here.\n(You can make a copy of, or modify, this frame)"
            n137 = Unbundle By Name(w370) -> ("RemoteControl out"=w367:refnum<class "RemoteControl.lvclass">)
            n138 = call-dynamic "Open Client Connection.vi"("error in (no error)"=w366, "RemoteControl in"=w367) -> ("error out"=w365:errorcluster, "RemoteControl out"=w368:refnum<class "RemoteControl.lvclass">)  [unwired: 8 in]
            n139 = Bundle By Name(cluster=w370, "RemoteControl out"=w368) -> (w369:T6)
            n140 = call <vilib>:"Add State(s) to Queue__JKI_lib_State_Machine.vi"("State(s) in (\"\")"=w373) -> ("States Out"=w372:string)  [unwired: 14 in]
          }
          frame "Client: Write" {
            # "Your code here.\n(You can make a copy of, or modify, this frame)"
            n141 = Unbundle By Name(w382) -> ("RemoteControl out"=w380:refnum<class "RemoteControl.lvclass">)
            n142 = local read "Message to Send"() -> (w377:T1)
            n143 = call <userlib>:"Wait (ms)__ogtk.vi"("error in (no error)"=w376, "milliseconds to wait"=u32 100) -> ("error out"=w375:errorcluster)  [unwired: 8 in, 1 out]
            n144 = call-dynamic "Send Message.vi"("error in (no error)"=w375, "Message"=w377, "RemoteControl in"=w380) -> ("error out"=w378:errorcluster, "RemoteControl out"=w379:refnum<class "RemoteControl.lvclass">)  [unwired: 7 in]
            n145 = Bundle By Name(cluster=w382, "RemoteControl out"=w379) -> (w381:T6)
            n146 = call <vilib>:"Add State(s) to Queue__JKI_lib_State_Machine.vi"("State(s) in (\"\")"=w385) -> ("States Out"=w384:string)  [unwired: 14 in]
          }
          frame "Client: Read" {
            # "Your code here.\n(You can make a copy of, or modify, this frame)"
            n147 = Unbundle By Name(w393) -> ("RemoteControl out"=w391:refnum<class "RemoteControl.lvclass">)
            n148 = while {
              tunnel: w391 -> [w409]
              tunnel: [w408] -> w390
              tunnel: "timeout in ms (100)" -> [w407]
              tunnel: [w402] -> w386
              tunnel: w388 -> [w406]
              tunnel: [w405] -> w387
              i -> [w404]
              stop <- w397 stop-if-true
              n149 = Greater?(x=w404, y=100) -> (0:w399:bool)
              n150 = call-dynamic "Read Message.vi"("timeout in ms (100)"=w407, "error in (no error)"=w406, "RemoteControl in"=w409) -> ("error out"=w405:errorcluster, "Message"=w402:T1, "RemoteControl out"=w408:refnum<class "RemoteControl.lvclass">)  [unwired: 5 in, 1 out]
              n151 = Unbundle By Name(w402) -> ("Command"=w401:string)
              n152 = Empty String/Path?(string/path=w401) -> (empty?=w400:bool)
              n153 = Not(x=w400) -> (.not. x?=w398:bool)
              n154 = Or(x=w398, y=w399) -> (x .or. y?=w397:bool)
              "# reads" <- w404
            }
            n155 = local write "Message Received"(w386) -> ()
            n156 = Bundle By Name(cluster=w393, "RemoteControl out"=w390) -> (w392:T6)
            n157 = call <vilib>:"Add State(s) to Queue__JKI_lib_State_Machine.vi"("State(s) in (\"\")"=w396) -> ("States Out"=w395:string)  [unwired: 14 in]
          }
          frame "Client: Close" {
            # "Your code here.\n(You can make a copy of, or modify, this frame)"
            n158 = Unbundle By Name(w415) -> ("RemoteControl out"=w413:refnum<class "RemoteControl.lvclass">)
            n159 = call-dynamic "Close Connection.vi"("error in (no error)"=w412, "RemoteControl in"=w413) -> ("error out"=w410:errorcluster, "RemoteControl out"=w411:refnum<class "RemoteControl.lvclass">)  [unwired: 8 in]
            n160 = Bundle By Name(cluster=w415, "RemoteControl out"=w411) -> (w414:T6)
            n161 = call <vilib>:"Add State(s) to Queue__JKI_lib_State_Machine.vi"("State(s) in (\"\")"=w418) -> ("States Out"=w417:string)  [unwired: 14 in]
          }
        }
      }
    }
    frame Enabled {
      w435 = refnum<class "RemoteControl.lvclass"> refnum  # RC (parent)
      w423 = refnum<class "RemoteControl.STM.lvclass"> refnum  # RC (child)
      # "this is a trick to make this VI able to access the child's methods\nthis VI shoudl actually be a part of the child class"
      n162 = Select(t=w423, s=TRUE, f=w435) -> (s? t:f=w422:refnum<class "RemoteControl.lvclass">)
      n163 = call-dynamic "Write Port.vi"("error in (no error)"=w425, "Port"=u32 6341, "RemoteControl in"=w422) -> ("error out"=w427:errorcluster, "RemoteControl out"=w428:refnum<class "RemoteControl.lvclass">)  [unwired: 7 in]
      n164 = call-dynamic "Open Client Connection.vi"("error in (no error)"=w427, "RemoteControl in"=w428) -> ("error out"=w421:errorcluster, "RemoteControl out"=w429:refnum<class "RemoteControl.lvclass">)  [unwired: 8 in]
      n165 = local read "Message to Send"() -> (w430:T1)
      n166 = call <userlib>:"Wait (ms)__ogtk.vi"("error in (no error)"=w421, "milliseconds to wait"=u32 0) -> ("error out"=w420:errorcluster)  [unwired: 8 in, 1 out]
      n167 = call-dynamic "Send Message.vi"("error in (no error)"=w420, "Message"=w430, "RemoteControl in"=w429) -> ("error out"=w431:errorcluster, "RemoteControl out"=w432:refnum<class "RemoteControl.lvclass">)  [unwired: 7 in]
      n168 = while {
        shift-right: [w449] -> w434
        shift-left: w432 -> [w447]
        shift-right: [w448] -> w433
        shift-left: w431 -> [w446]
        i -> [w440]
        stop <- w441 stop-if-true
        n169 = local write "# reads"(w440) -> ()
        n170 = Greater?(x=w440, y=20) -> (0:w442:bool)
        n171 = call-dynamic "Read Message.vi"("timeout in ms (100)"=100, "error in (no error)"=w446, "RemoteControl in"=w447) -> ("error out"=w448:errorcluster, "Message"=w438:T1, "RemoteControl out"=w449:refnum<class "RemoteControl.lvclass">)  [unwired: 5 in, 1 out]
        n172 = local write "Message Received"(w438) -> ()
        n173 = Unbundle By Name(w438) -> ("Command"=w444:string)
        n174 = Empty String/Path?(string/path=w444) -> (empty?=w443:bool)
        n175 = Not(x=w443) -> (.not. x?=w437:bool)
        n176 = Or(x=w437, y=w442) -> (x .or. y?=w441:bool)
      }
      n177 = call-dynamic "Close Connection.vi"("error in (no error)"=w433, "RemoteControl in"=w434) -> ("error out"=w424:errorcluster)  [unwired: 8 in, 1 out]
    }
  }
  n178 = call <userlib>:"Tick Count (ms)__ogtk.vi"("error in (no error)"=w2) -> ("error out"=→"error out":errorcluster, "millisecond timer value"=w5:u32)  [unwired: 9 in]
  n179 = Subtract(x=w5, y=w1) -> (x-y=→"execution time (ms)":u32)
